vi "_jki-json_Marshal.vi"   [LabVIEW 2013, in "OpenSerializer.JKI-JSON.lvlib"]
uses:
  OpenSerializer.JKI-JSON.lvlib
  <vilib>/LabVIEW Open Source Project/OpenSerializer/Serializer/Serializer.lvclass
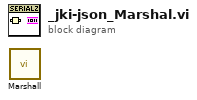
[diagram p0: block diagram]
diagram:
  n1 = call <vilib>:"Marshall.vi"() -> ()  [unwired: 9 in, 3 out]
